vi "Scripting Constants.vi"() -> ()   [LabVIEW 2017, in "Switch Scripting.lvlib"]
doc: "Use this Global VI to access the GUIDs assigned to the page resources of the Custom Device."
uses:
  Switch Scripting.lvlib
panel:
  in  "Tab Control":enum32{"GUIDS", "Constants", "Properties"}(tab)
  in  "RAF:CD:GUID":string="4e591626-626d-4903-9a6e-1f2a7b879f4d"
  in  "RAF:Channel:Descriptions":string="Descriptions"
  in  "RAF:State:Description":string="_Description"
  in  "RAF:State:DefaultValue":i32
  in  "RAF:State:DefaultName":string="Default"
  in  "RAF:Routes":string="Routes"
  in  "RAF:Aliases":string="Aliases"
  in  "RAF:Channel:Connections":string="Connections"
  in  "RAF:Name":string="Routing and Faulting Custom Device"
  in  "Compiled.Settings":string="Compiled.Settings"
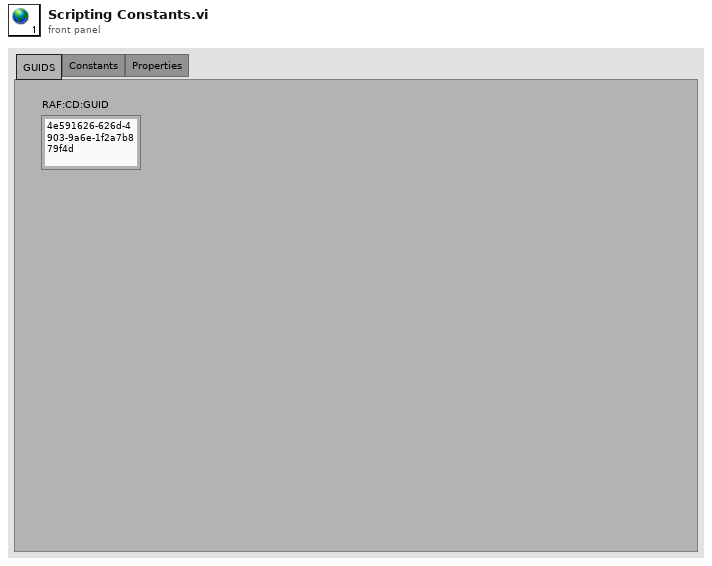
[diagram p1: front panel]
diagram:
